vi "TEST - Format Numeric Array.vi"(8 "error in (no error)":errorcluster) -> (0 "error out":errorcluster, 2 "pass":bool)   [LabVIEW 2020, in "test_openg_variant_config_file.lvlib"]
uses:
  <vilib>/addons/_JKI Toolkits/Caraya/classes/Assert/Assert True.vi
  test_openg_variant_config_file.lvlib
  source/library/openg_variant_configuration_file.lvlib
  <vilib>/addons/_JKI Toolkits/Caraya/classes/Test/Test.lvclass
  <vilib>/addons/_JKI Toolkits/Caraya/classes/Assert/Assert.lvclass
panel:
  out "Failures":T1(array[cluster]) {"input"."Array" format="%.2f"}
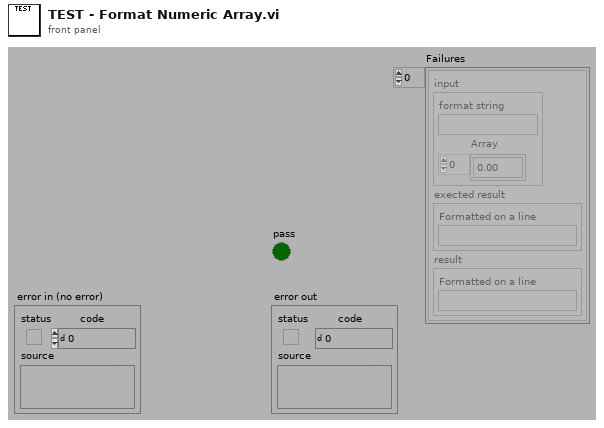
[diagram p1: front panel]
types:
  T1 = cluster{"input":cluster{"format string":string, "Array":dbl[]}, "exected result":cluster{"Formatted on a line":string}, "result":cluster{"Formatted on a line":string}}[]
  T2 = cluster{"input":cluster{"format string":string, "Array":dbl[]}, "exected result":cluster{"Formatted on a line":string}, "result":cluster{"Formatted on a line":string}}
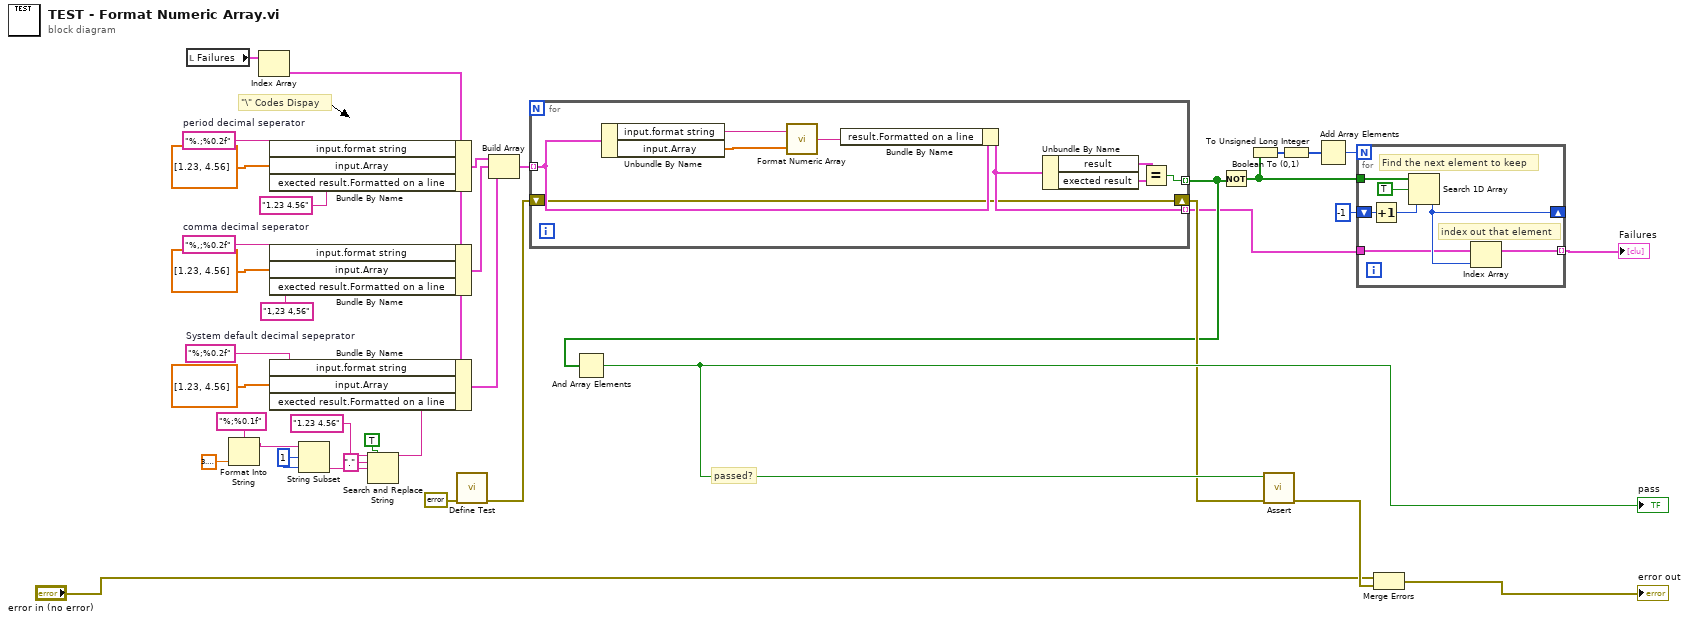
[diagram p0: block diagram]
diagram:
  w12 = 1 ("offset (0)")
  w14 = "%;%0.2f"  # System default decimal sepeprator
  w17 = "%,;%0.2f"  # comma decimal seperator
  w20 = "%.;%0.2f"  # period decimal seperator
  # "\"\\\" Codes Dispay"
  # "passed?"
  n1 = local read "Failures"() -> (w22:T1)
  n2 = Format Into String(format string="%;%0.1f", 3.141592653589793) -> (resulting string=w11:string)  [unwired: 2 in, 1 out]
  n3 = Index Array(array=w22) -> (element=w3:T2)  [unwired: 1 in]
  n4 = Bundle By Name(cluster=w3, "input.format string"=w20, "input.Array"=dbl[] [1.23, 4.56], "exected result.Formatted on a line"="1.23 4.56") -> (w24:T2)
  n5 = Bundle By Name(cluster=w3, "input.format string"=w17, "input.Array"=dbl[] [1.23, 4.56], "exected result.Formatted on a line"="1,23 4,56") -> (w15:T2)
  n6 = String Subset(string=w11, offset (0)=w12, length (rest)=w12) -> (substring=w6:string)
  n7 = Search and Replace String(replace all?=TRUE ("replace all? (F)"), input string="1.23 4.56" ("exected result.Formatted on a line"), search string=".", replace string=w6) -> (result string=w4:string)  [unwired: 4 in, 3 out]
  n8 = Bundle By Name(cluster=w3, "input.format string"=w14, "input.Array"=dbl[] [1.23, 4.56], "exected result.Formatted on a line"=w4) -> (w2:T2)
  n9 = call <vilib>:"Define Test.vi"("error in (no error)"=errorcluster {"status"=FALSE, "code"=0, "source"=""}) -> ("error out"=w35:errorcluster)  [unwired: 9 in, 1 out]
  n10 = Build Array(w24, w15, w2) -> (w23:T1)
  n11 = for {
    tunnel: w23 -> [w46] mode=indexing
    tunnel: [w47] -> w26 mode=indexing
    tunnel: [w45] -> w25 mode=indexing
    shift-right: [w42] -> w33
    shift-left: w35 -> [w42]
    n12 = Unbundle By Name(w46) -> ("input.format string"=w41:string, "input.Array"=w40:dbl[])
    n13 = call "Format Numeric Array.vi"("Array"=w40, "format string"=w41) -> ("Formatted on a line"=w39:string)
    n14 = Bundle By Name(cluster=w46, "result.Formatted on a line"=w39) -> (w45:T2)
    n15 = Unbundle By Name(w45) -> ("result"=w44:cluster{"Formatted on a line":string}, "exected result"=w43:cluster{"Formatted on a line":string})
    n16 = Equal?(x=w44, y=w43) -> (x = y?=w47:bool)
  }
  n17 = And Array Elements(Boolean array=w26) -> (logical AND=w34:bool)
  "pass" <- w34
  n18 = Not(x=w26) -> (.not. x?=w28:bool[])
  n19 = Boolean To (0,1)(Boolean=w28) -> (0, 1=w29:i16[])
  n20 = call-poly <vilib>:"Assert.vi"("error in (no error)"=w33, "True?"=w34) -> ("error out"=w32:errorcluster)  [unwired: 8 in, 1 out]
  n21 = To Unsigned Long Integer(number=w29) -> (unsigned 32bit integer=w27:u32[])
  n22 = Add Array Elements(numeric array=w27) -> (sum=w30:u32)
  n23 = for {
    N: w30 -> [_]
    tunnel: w25 -> [w50]
    tunnel: w28 -> [w54]
    shift-right: [w51] -> _
    shift-left: -1 ("start index (0)") -> [w52]
    tunnel: [w49] -> w37 mode=indexing
    # "index out that element"
    # "Find the next element to keep"
    n24 = Increment(x=w52) -> (x+1=w48:i32)
    n25 = Search 1D Array(1D array=w54, element=TRUE, start index (0)=w48) -> (index of element=w51:i32)
    n26 = Index Array(array=w50, index=w51) -> (element=w49:T2)
  }
  "Failures" <- w37
  n27 = Merge Errors("error in (no error)", w32) -> (→"error out":errorcluster)
